vi "SaveAlarms.vi"(8 "error in (no error)":errorcluster, 9 "data flow":T9, 11 "data event":T1) -> (0 "error out":errorcluster, 3 "data event out":T1)   [LabVIEW 2017, in "DataEventCreator.lvlib"]
uses:
  <vilib>/addons/InsightCM/Devices/Shared/Common/DataEventCreator/DataEventCreator.lvlib
  <vilib>/addons/InsightCM/Devices/Shared/Common/DataFlow/controls/Data.ctl
  <vilib>/addons/InsightCM/Utilities/DataAccessors/controls/wfmSGL_DVR.ctl
  <vilib>/addons/PointValueMap/controls/PointMap.ctl
  <vilib>/addons/InsightCM/Devices/Shared/Common/DataFlow/controls/Type.ctl
  <vilib>/addons/InsightCM/Devices/Shared/Common/DataEvent/controls/Event.ctl
  <vilib>/addons/InsightCM/MessageBus/Base/controls/DataEvent.ctl
  <vilib>/addons/InsightCM/MessageBus/Base/controls/KeyValuePair.ctl
  <vilib>/addons/InsightCM/Devices/Shared/Common/DataEvent/controls/DataSet.ctl
  <vilib>/addons/InsightCM/MessageBus/Base/controls/DataSetMetadata.ctl
  <vilib>/addons/InsightCM/MessageBus/Base/controls/TrendPoint.ctl
  <vilib>/addons/InsightCM/MessageBus/Base/controls/TrendAlarmUpdate.ctl
  <vilib>/addons/InsightCM/MessageBus/Base/controls/TrendAlarmTransition.ctl
  <vilib>/addons/PointValueMap/subVIs/Point_Read_variant.vi
  <vilib>/addons/PointValueMap/PointValueMap.lvlib
  <vilib>/addons/InsightCM/Devices/Shared/Common/DataEvent/DataEvent.lvlib
  <vilib>/addons/InsightCM/Devices/Shared/Common/DataFlow/DataFlow.lvlib
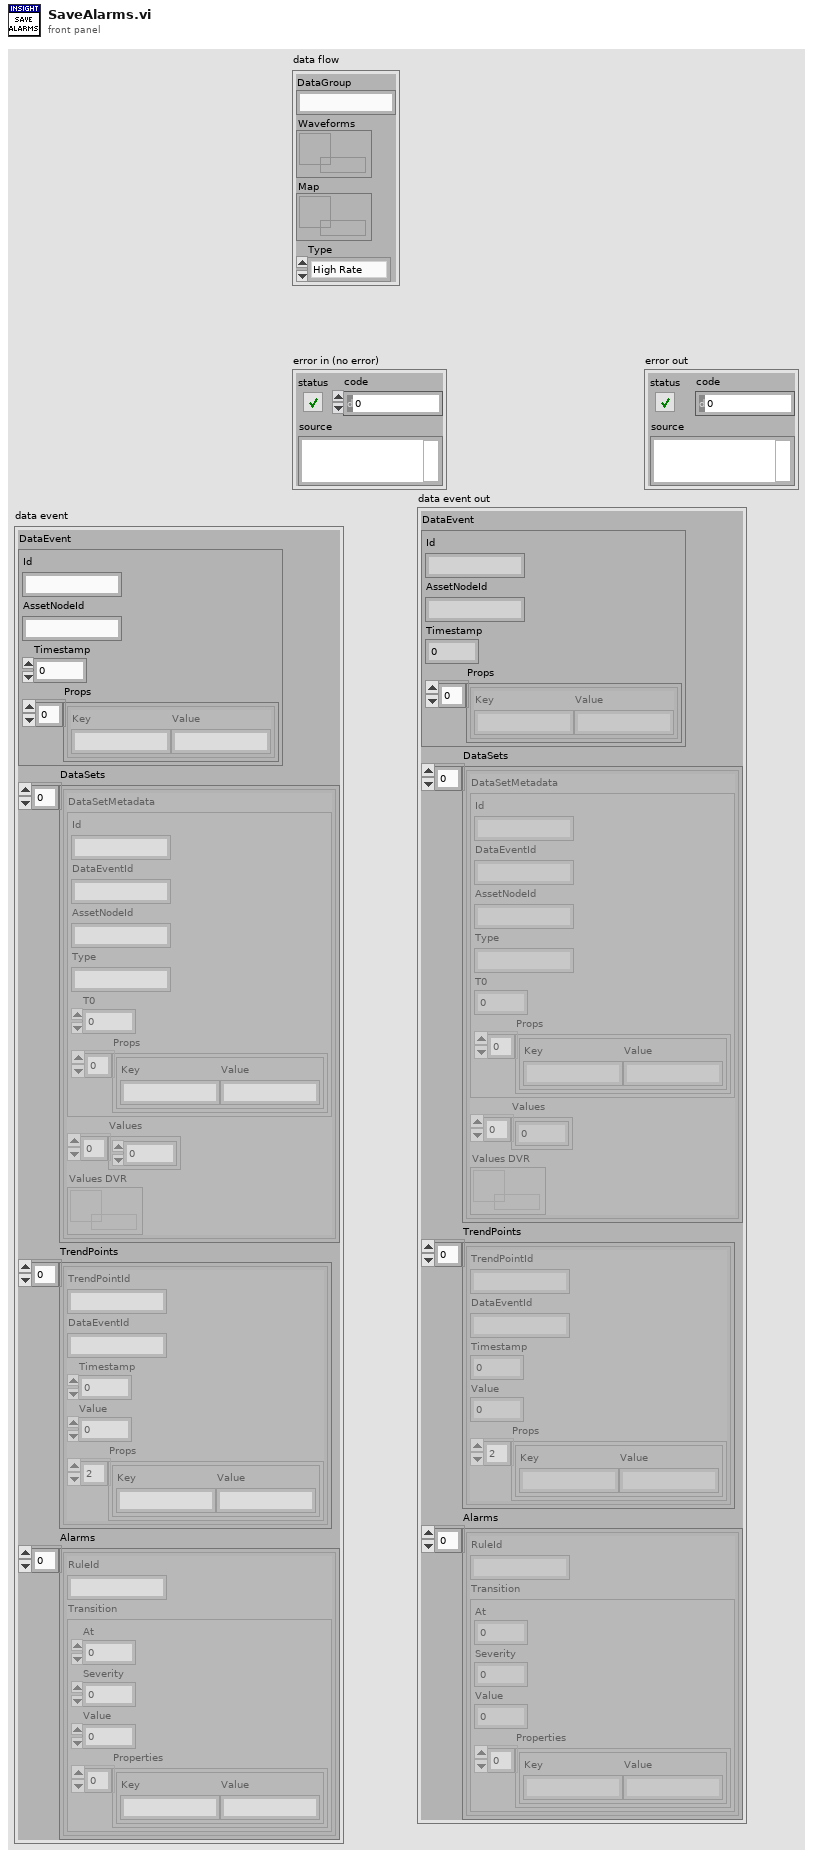
[diagram p1: front panel]
types:
  T1 = typedef "DataEvent.lvlib/Event.ctl" = cluster{"DataEvent":T2, "DataSets":T4[], "TrendPoints":T6[], "Alarms":T7[]}
  T2 = typedef "DataEvent.ctl" = cluster{"Id":string, "AssetNodeId":string, "Timestamp":i64, "Props":T3[]}
  T3 = typedef "KeyValuePair.ctl" = cluster{"Key":string, "Value":string}
  T4 = typedef "DataEvent.lvlib/DataSet.ctl" = cluster{"DataSetMetadata":T5, "Values":sgl[], "Values DVR":refnum<data-value>}
  T5 = typedef "DataSetMetadata.ctl" = cluster{"Id":string, "DataEventId":string, "AssetNodeId":string, "Type":string, "T0":i64, "Props":T3[]}
  T6 = typedef "TrendPoint.ctl" = cluster{"TrendPointId":string, "DataEventId":string, "Timestamp":i64, "Value":dbl, "Props":T3[]}
  T7 = typedef "TrendAlarmUpdate.ctl" = cluster{"RuleId":string, "Transition":T8}
  T8 = typedef "TrendAlarmTransition.ctl" = cluster{"At":i64, "Severity":i32, "Value":dbl, "Properties":T3[]}
  T9 = typedef "DataFlow.lvlib/Data.ctl" = cluster{"DataGroup":string, "Waveforms":T10, "Map":T11, "Type":T12}
  T10 = typedef "wfmSGL_DVR.ctl" = refnum<data-value>
  T11 = typedef "PointValueMap.lvlib/PointMap.ctl" = refnum<data-value>
  T12 = typedef "DataFlow.lvlib/Type.ctl" = enum16{"High Rate", "Low Rate", "Burst Mode"}
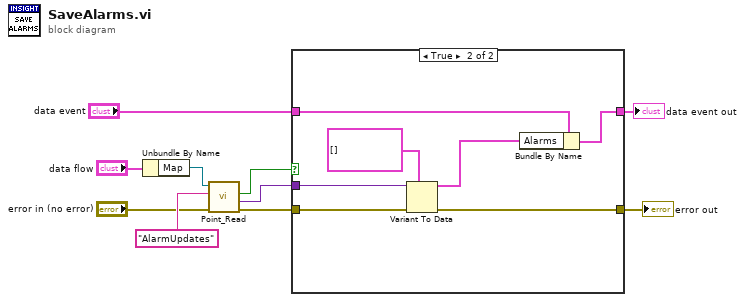
[diagram p0: block diagram]
diagram:
  n1 = Unbundle By Name("data flow") -> ("Map"=w3:T11)
  n2 = call-poly <vilib>:"Point_Read.vi"("Error In"="error in (no error)", "Tag"="AlarmUpdates", "Map"=w3) -> ("Error Out"=w7:errorcluster, "Value"=w6:variant, "Found?"=w5:bool)  [unwired: 3 in, 3 out]
  n3 = case shown="True" w5 {
    tunnel: [w12 w19] -> w10
    tunnel: w7 -> [w12 w18]
    tunnel: w6 -> [_ w17]
    tunnel: "data event" -> [w11 w16]
    tunnel: [w11 w13] -> w1
    frame False {
    }
    frame True {
      n4 = Variant To Data(error in=w18, type=T7[] [], Variant=w17) -> (data=w14:T7[], error out=w19:errorcluster)
      n5 = Bundle By Name(cluster=w16, "Alarms"=w14) -> (w13:T1)
    }
  }
  "error out" <- w10
  "data event out" <- w1
